vi "Rename Class Controls.vi"(6 "Old Class":path, 8 "error in":errorcluster, 9 "Class To Rename":refnum<vi>, 10 "Application Instance":refnum<vi>) -> (0 "error out":errorcluster)   [LabVIEW 2021, in "_Rename.lvlib" / "_Rename.lvclass"]
uses:
  Script/_Rename.lvclass
  <vilib>/Utility/traverseref.llb/TRef TravTarget.ctl
  Script/_Rename.lvclass/_Rename.ctl
  <vilib>/Utility/traverseref.llb/VI Scripting - Traverse.lvlib
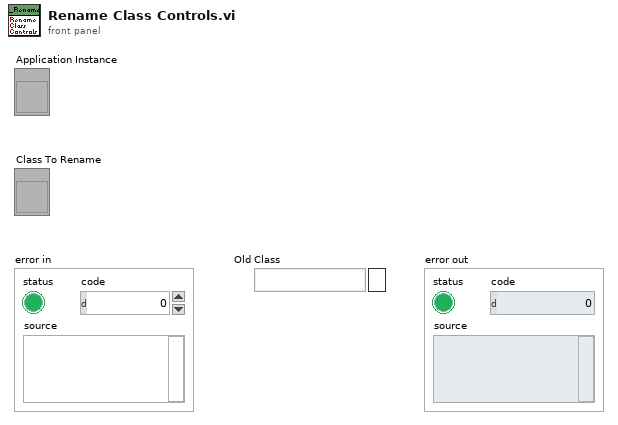
[diagram p1: front panel]
types:
  T1 = typedef "TRef TravTarget.ctl" = enum16{"FP", "BD", "Other"}
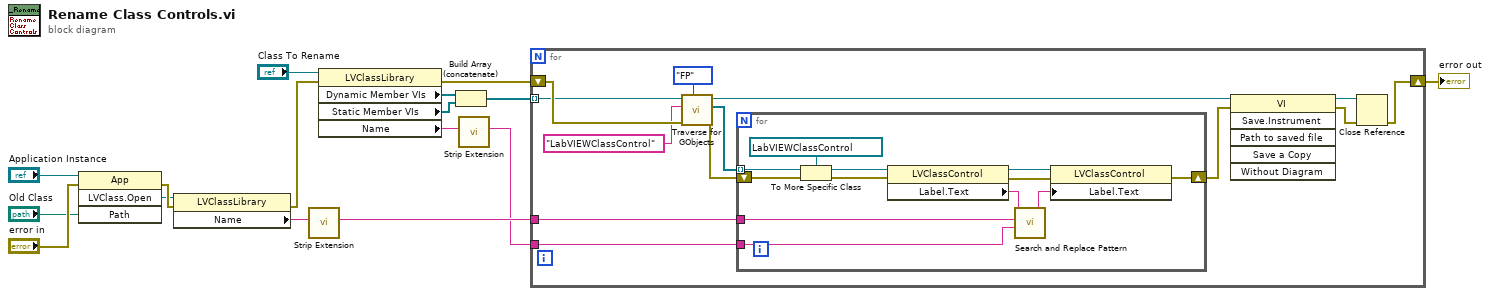
[diagram p0: block diagram]
diagram:
  n1 = invoke class="App" method="LVClass.Open"(reference="Application Instance", error in="error in", "Path"="Old Class") -> (error out=w15:errorcluster, "LVClass.Open"=w10:refnum<vi>)  [unwired: 1 in, 2 out]
  n2 = property class="LVClassLibrary"(reference=w10, error in=w15) -> (error out=w16:errorcluster, "Name"=w4:string)  [unwired: 1 out]
  n3 = call "Strip Extension.vi"("Name with Extension"=w4) -> ("Name without Extension"=w3:string)  [unwired: 10 in]
  n4 = property class="LVClassLibrary"(reference="Class To Rename", error in=w16) -> (error out=w13:errorcluster, "Dynamic Member VIs"=w6:refnum<vi>[], "Static Member VIs"=w7:refnum<vi>[], "Name"=w2:string)  [unwired: 1 out]
  n5 = Build Array (concatenate)(w6, w7) -> (w8:refnum<vi>[])
  n6 = call "Strip Extension.vi"("Name with Extension"=w2) -> ("Name without Extension"=w1:string)  [unwired: 10 in]
  n7 = for {
    tunnel: w8 -> [w24] mode=indexing
    tunnel: w1 -> [w17]
    tunnel: w3 -> [w20]
    shift-right: [w25] -> w12
    shift-left: w13 -> [w29]
    n8 = call <vilib>:"Traverse for GObjects.vi"("Traverse Target"=TRef_TravTarget."FP", "error in (no error)"=w29, "Class Name"="LabVIEWClassControl", "VI Refnum"=w24) -> ("error out"=w28:errorcluster, "References"=w21:refnum<vi>[], "dup VI Refnum"=w18:refnum<vi>)  [unwired: 4 in, 1 out]
    n9 = for {
      tunnel: w21 -> [w37] mode=indexing
      tunnel: w17 -> [w33]
      tunnel: w20 -> [w31]
      shift-right: [w38] -> w27
      shift-left: w28 -> [w39]
      n10 = To More Specific Class(target class=refnum<vi> refnum ("LVClassControl Refnum"), reference=w37, error in=w39) -> (specific class reference=w36:refnum<vi>, error out=w41:errorcluster)
      n11 = property class="LVClassControl"(reference=w36, error in=w41) -> (reference out=w35:refnum<vi>, error out=w40:errorcluster, "Label.Text"=w34:string)
      n12 = call <vilib>:"Search and Replace Pattern.vi"("string"=w34, "regular expression (\"\")"=w31, "replace string (\"\")"=w33) -> ("result string"=w32:string)  [unwired: 2 in, 1 out]
      n13 = property class="LVClassControl"(reference=w35, error in=w40, "Label.Text"=w32) -> (error out=w38:errorcluster)  [unwired: 1 out]
    }
    n14 = invoke class="VI" method="Save.Instrument"(reference=w18, error in=w27) -> (reference out=w19:refnum<vi>, error out=w26:errorcluster)  [unwired: 4 in, 4 out]
    n15 = Close Reference(reference=w19, error in (no error)=w26) -> (error out=w25:errorcluster)
  }
  "error out" <- w12
